vi "pre-chirper comms.vi"() -> ()   [LabVIEW 2020]
doc: "This example performs a serial port write and a serial port read. The parameters set for the serial port must match the parameters of the connected instrument or device. The VISA Configure Serial Port VI sets the configuration parameters. The front panel displays the controls used to configure the basic parameters, such as baud rate, data bits, and parity. The VI passes the VISA resource name to other VIs that perform operations on that VISA resource. The VISA Write function sends a command to the serial device and the VISA Read function returns data based on the command. The VISA Close function then closes the reference to the serial device. It is important to close the reference; otherwise, further communication through that port might not be possible."
uses:
  <vilib>/Instr/_visa.llb/VISA Configure Serial Port (Instr).vi
panel:
  out "Write return count":u32
  out "length":i32
  in  "Command":string="#E00000000"
  in  "delay before read (ms)":u32=50
  in  "flow control":u16(ring) items=["None"=0, "XON/XOFF"=1, "RTS/CTS"=2, "DTR/DSR"=4]
  in  "stop bits":u16(ring)=10 items=["1.0"=10, "1.5"=15, "2.0"=20]
  in  "parity":enum16{"None", "Odd", "Even", "Mark", "Space"}(ring)
  in  "data bits":u16=8 min=5 max=8 step=1
  in  "baud rate":u32(ring)=19200 items=["75"=75, "110"=110, "134"=134, "150"=150, "300"=300, "600"=600, "1200"=1200, "1800"=1800, "2400"=2400, "4800"=4800, "7200"=7200, "9600"=9600, "14400"=14400, "19200"=19200, "28800"=28800, "38400"=38400, "56000"=56000, "57600"=57600, "115200"=115200, "128000"=128000, "230400"=230400]
  in  "VISA resource name":refnum<visa-resource-name>="COM11"
  out "hex integer string":string[](array[string])
  out "error out":errorcluster
  out "Read return count":u32
  out "bytes read":u32
  out "Response":string
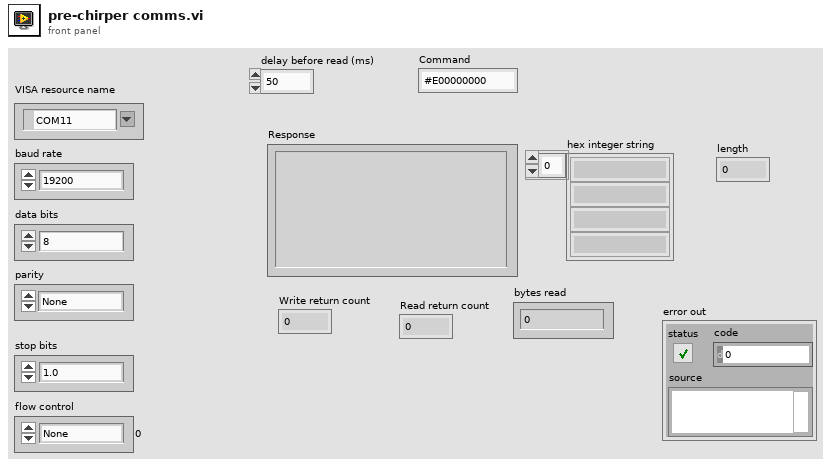
[diagram p1: front panel]
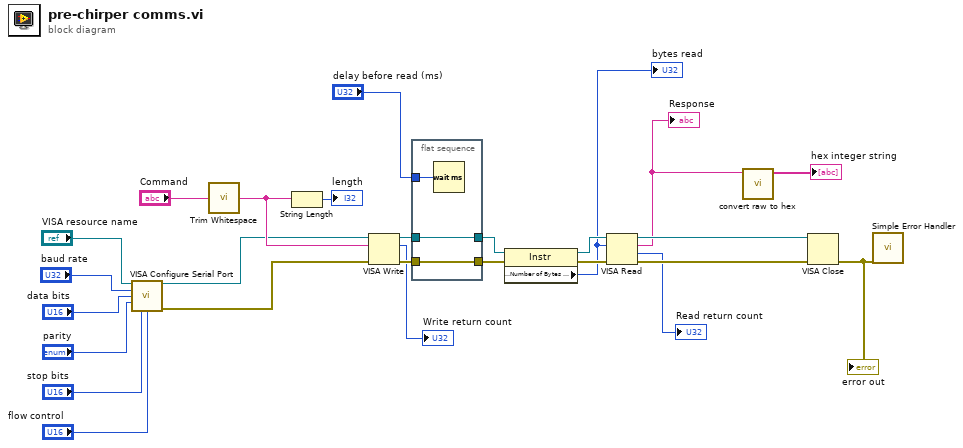
[diagram p0: block diagram]
diagram:
  n1 = call-poly "VISA Configure Serial Port"("VISA resource name"="VISA resource name", "baud rate (9600)"="baud rate", "data bits (8)"="data bits", "parity (0:none)"="parity", "stop bits (10: 1 bit)"="stop bits", "flow control (0:none)"="flow control") -> ("VISA resource name out"=w1:refnum<visa-resource-name>, "error out"=w2:errorcluster)  [unwired: 3 in, 5 out]
  n2 = call <vilib>:"Trim Whitespace.vi"("string"="Command") -> ("trimmed string"=w5:string)  [unwired: 1 in]
  n3 = String Length(string=w5) -> (length=→"length":i32)
  n4 = VISA Write(VISA resource name=w1, write buffer=w5, error in (no error)=w2) -> (VISA resource name out=w21:refnum<visa-resource-name>, return count=→"Write return count":u32, error out=w23:errorcluster)
  n5 = flat-sequence {
    tunnel: w23 -> [w28]
    tunnel: [w28] -> w22
    tunnel: w21 -> [w27]
    tunnel: [w27] -> w20
    tunnel: "delay before read (ms)" -> [w29]
    frame #0 {
      n6 = Wait (ms)(milliseconds to wait=w29) -> ()  [unwired: 1 out]
    }
  }
  n7 = property class="Instr"(reference=w20, error in=w22) -> (reference out=w19:refnum<visa-resource-name>, error out=w18:errorcluster, "Serial Settings:Number of Bytes at Serial Port"=w17:u32)
  "bytes read" <- w17
  n8 = VISA Read(VISA resource name=w19, byte count=w17, error in (no error)=w18) -> (VISA resource name out=w25:refnum<visa-resource-name>, read buffer=w15:string, return count=→"Read return count":u32, error out=w26:errorcluster)
  "Response" <- w15
  n9 = call "convert raw to hex.vi"("String"=w15) -> ("hex integer string"=→"hex integer string":string[])  [unwired: 10 in]
  n10 = VISA Close(VISA resource name=w25, error in (no error)=w26) -> (error out=w24:errorcluster)
  "error out" <- w24
  n11 = call <vilib>:"Simple Error Handler.vi"("error in (no error)"=w24) -> ()  [unwired: 1 in, 8 out]
